vi "MakeCustomWindow (SubVI).vi"(9 "radialaxis":dbl[](array[numeric])=[0.0, 1.0, 2.0, 3.0, 4.0, 5.0, 6.0, 7.0, 8.0, 9.0, 10.0, 11.0, 12.0, 13.0, 14.0, 15.0, 16.0, 17.0, 18.0, 19.0, 20.0]) -> (1 "Stetson":dbl[](graph), 2 "hamming":dbl[](graph), 3 "Halfstetson":dbl[](graph))   [LabVIEW 2011, in "OfflineTracker.lvlib"]
uses:
  <vilib>/Analysis/4window.llb/Hamming Window (DBL).vi
  OfflineTracker.lvlib
  <vilib>/Analysis/NI_AALPro.lvlib
panel:
  in  "rise":dbl=5.0
  in  "fall":dbl=1.0
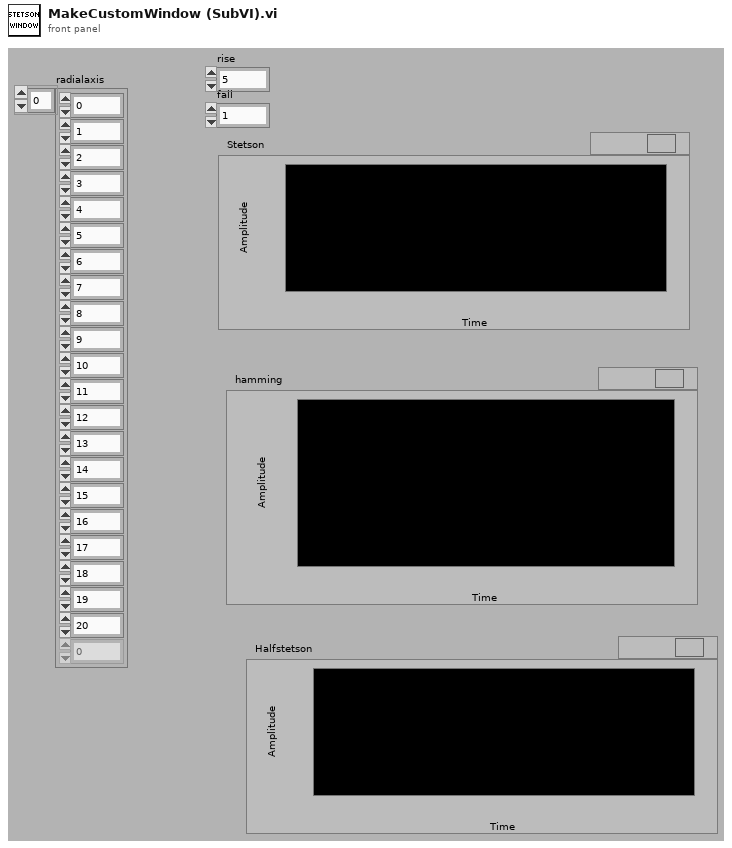
[diagram p1: front panel]
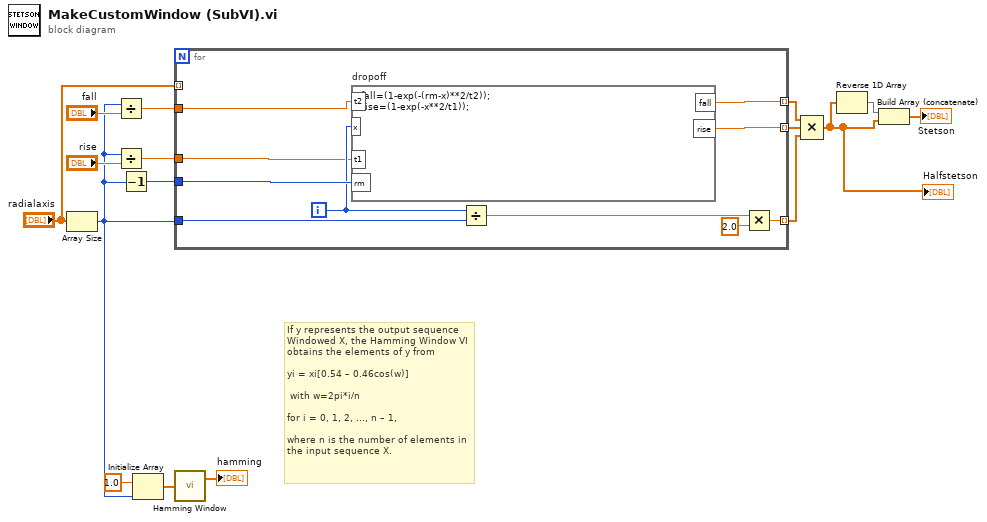
[diagram p0: block diagram]
diagram:
  # "If y represents the output sequence Windowed X, the Hamming Window VI obtains the elements of y from\n\nyi = xi[0.54 – 0.46cos(w)]\n\n with w=2pi*i/n\n\nfor i = 0, 1, 2, …, n – 1,\n\nwhere n is the number of elements in the input sequence X."
  n1 = Array Size(array="radialaxis") -> (size(s)=w3:i32)
  n2 = Divide(x=w3, y="fall") -> (x/y=w13:dbl)
  n3 = Divide(x=w3, y="rise") -> (x/y=w14:dbl)
  n4 = Decrement(x=w3) -> (x-1=w2:i32)
  n5 = Initialize Array(1.0 ("element"), w3) -> (w11:dbl[])
  n6 = for {
    tunnel: w14 -> [w18]
    tunnel: "radialaxis" -> [_] mode=indexing
    tunnel: [w17] -> w8 mode=indexing
    tunnel: w13 -> [w24]
    tunnel: w2 -> [w26]
    tunnel: [w25] -> w9 mode=indexing
    tunnel: w3 -> [w22]
    tunnel: [w19] -> w7 mode=indexing
    i -> [w21]
    n7 = formula code="fall=(1-exp(-(rm-x)**2/t2));\nrise=(1-exp(-x**2/t1));" "dropoff"("x"=w21, "t2"=w24, "rm"=w26, "t1"=w18) -> ("fall"=w25:dbl, "rise"=w17:dbl)
    n8 = Divide(x=w21, y=w22) -> (x/y=w20:dbl)
    n9 = Multiply(x=w20, y=2.0) -> (x*y=w19:dbl)
  }
  n10 = call-poly <vilib>:"Hamming Window.vi"("X"=w11) -> ("Windowed X"=→"hamming":dbl[])  [unwired: 1 out]
  n11 = Compound Arithmetic op=MULTIPLY(w9, w8, w7) -> (w1:dbl[])
  "Halfstetson" <- w1
  n12 = Reverse 1D Array(array=w1) -> (reversed array=w6:dbl[])
  n13 = Build Array (concatenate)(w6, w1) -> (→"Stetson":dbl[])
